vi "Configure Channel (Basic).vi"(5 "Impedance (1E+6 Ohm)":dbl(ring)=1000000.0 items=["50"=50.0, "1E+6"=1000000.0], 6 "Enable Noise Rejection (F: Disable)":bool, 7 "Enable Filter (F: Disable)":bool, 8 "error in (no error)":errorcluster, 9 "Coupling (0: AC)":i32(ring) items=["AC", "DC"], 10 "Channel (1: Channel 1)":i32(ring)=1 items=["Channel 1"=1, "Channel 2"=2], 11 "VISA resource name":refnum<visa-resource-name>) -> (0 "error out":errorcluster, 3 "VISA resource name out":refnum<visa-resource-name>)   [LabVIEW 2024, in "Agilent 532XX Series.lvlib"]
doc: "Configures the basic characteristics of the channel to which an input is connected."
uses:
  Agilent 532XX Series.lvlib
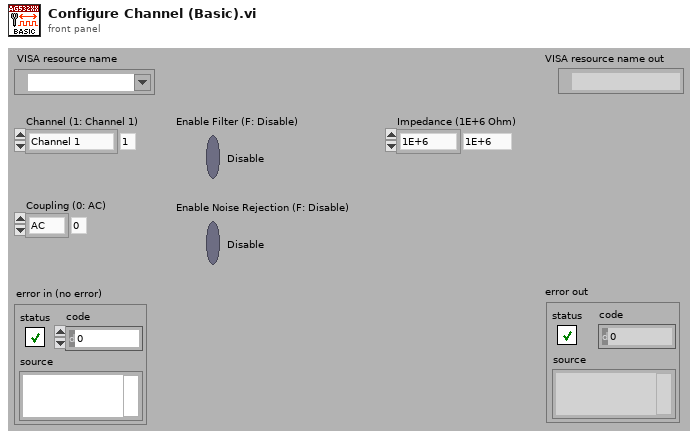
[diagram p1: front panel]
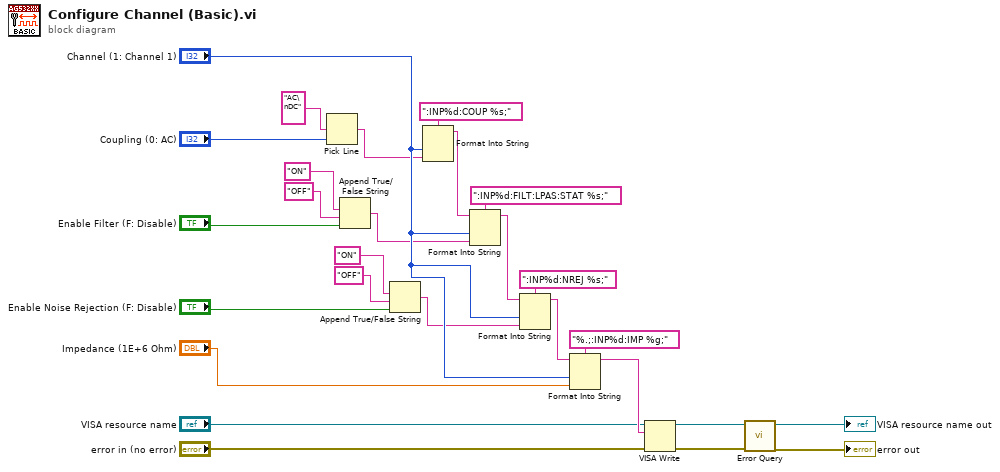
[diagram p0: block diagram]
diagram:
  n1 = Pick Line(multi-line string="AC\nDC", line index="Coupling (0: AC)") -> (output string=w23:string)  [unwired: 1 out]
  n2 = Append True/False String(1:"Enable Filter (F: Disable)", 2:"OFF", 3:"ON") -> (0:w17:string)  [unwired: 1 out]
  n3 = Append True/False String(1:"Enable Noise Rejection (F: Disable)", 2:"OFF", 3:"ON") -> (0:w11:string)  [unwired: 1 out]
  n4 = Format Into String(format string=":INP%d:COUP %s;", "Channel (1: Channel 1)", w23) -> (resulting string=w19:string)  [unwired: 2 in, 1 out]
  n5 = Format Into String(format string=":INP%d:FILT:LPAS:STAT %s;", initial string=w19, "Channel (1: Channel 1)", w17) -> (resulting string=w13:string)  [unwired: 1 in, 1 out]
  n6 = Format Into String(format string=":INP%d:NREJ %s;", initial string=w13, "Channel (1: Channel 1)", w11) -> (resulting string=w10:string)  [unwired: 1 in, 1 out]
  n7 = Format Into String(format string="%.;:INP%d:IMP %g;", initial string=w10, "Channel (1: Channel 1)", "Impedance (1E+6 Ohm)") -> (resulting string=w7:string)  [unwired: 1 in, 1 out]
  n8 = VISA Write(VISA resource name="VISA resource name", write buffer=w7, error in (no error)="error in (no error)") -> (VISA resource name out=w4:refnum<visa-resource-name>, error out=w3:errorcluster)  [unwired: 1 out]
  n9 = call "Error Query.vi"("error in (no error)"=w3, "VISA resource name"=w4) -> ("error out"=→"error out":errorcluster, "VISA resource name out"=→"VISA resource name out":refnum<visa-resource-name>)  [unwired: 8 out]
